vi "Create Success.vi"(5 "Test Case in":refnum<class "Test Case.lvclass">, 8 "error in (no error)":errorcluster, 9 "Time":dbl, 10 "Classname":string, 11 "Name":string) -> (0 "error out":errorcluster, 3 "Test Case":refnum<class "Test Case.lvclass">)   [LabVIEW 2013, in "JUnit XML.lvlib" / "Test Case.lvclass"]
uses:
  Test Case.lvclass
  Test Result.ctl
  Test Case.lvclass/Test Case.ctl
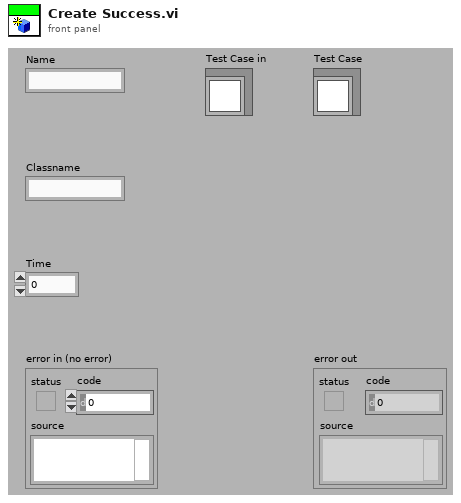
[diagram p1: front panel]
types:
  T1 = typedef "JUnit XML.lvlib/Test Case.lvclass/Test Result.ctl" = enum16{"Success", "Failure", "Error", "Skipped"}
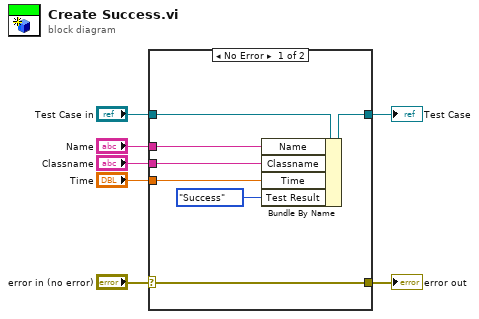
[diagram p0: block diagram]
diagram:
  n1 = case shown="No Error" "error in (no error)" {
    selector: "error in (no error)" -> [w14 w16]
    tunnel: [w14 w16] -> w6
    tunnel: [w12 w15] -> w4
    tunnel: "Test Case in" -> [w13 w15]
    tunnel: "Name" -> [w11 _]
    tunnel: "Classname" -> [w10 _]
    tunnel: "Time" -> [w9 _]
    frame No Error {
      n2 = Bundle By Name(cluster=w13, "Name"=w11, "Classname"=w10, "Time"=w9, "Test Result"=Test_Result."Success") -> (w12:refnum<class "Test Case.lvclass">)
    }
    frame Error {
    }
  }
  "error out" <- w6
  "Test Case" <- w4
